vi "Notifier-with-memory-boolean.vi"(8 "error in":errorcluster, 10 "Timeout [ms]":i32, 11 "Notifier in":refnum<notifier>) -> (0 "error IO":errorcluster, 2 "Notification":bool)   [LabVIEW 2013, in "CameraVision.lvlib" / "CV-UI.lvclass"]
doc: "Polymorphic type of Notifier-with-memory vi.\n\nAccepts a notifier reference for a single boolean.\nThe vi listens for 'Timeout' miliseconds for a new message on the notifier.\nIf no message arrives or arrived before calling the vi, the last received message is returned.\n\nThe default message is a false boolean."
uses:
  CV-UI.lvclass
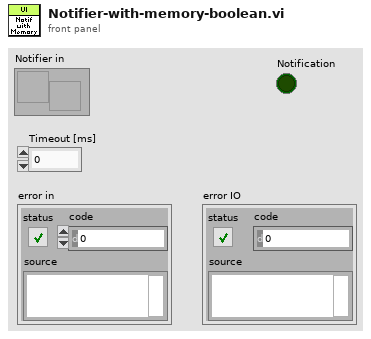
[diagram p1: front panel]
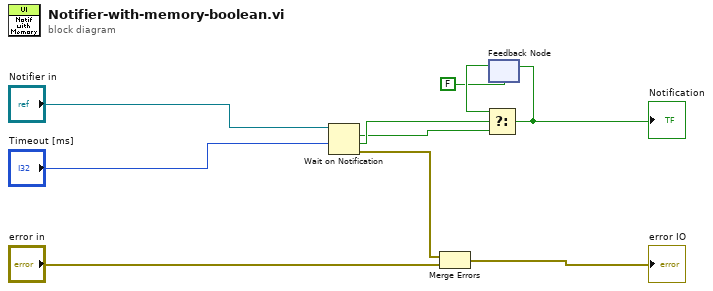
[diagram p0: block diagram]
diagram:
  n1 = Wait on Notification(notifier="Notifier in", timeout in ms (-1)="Timeout [ms]") -> (notification=w5:bool, timed out?=w6:bool, error out=w10:errorcluster)  [unwired: 2 in, 1 out]
  n2 = Merge Errors(w10, "error in") -> (→"error IO":errorcluster)
  n3 = feedback #1(FALSE) -> (w4:bool)
  n4 = Select(t=w4, s=w6, f=w5) -> (s? t:f=w7:bool)
  "Notification" <- w7
  n5 = feedback-in #1(w7) -> ()
